vi "PDC_AVIFileSave.vi"(8 "error in (no error)":errorcluster, 9 "FrameNo":u32, 10 "ChildNo":u32, 11 "DeviceNo":u32) -> (0 "error out":errorcluster, 2 "Size":u32, 3 "ReturnValue":u32, 4 "ErrorCode":u32)   [LabVIEW 2015]
doc: "Saves AVI files for specified images which recorded by the specified child device."
uses:
  PDCLIB.dll
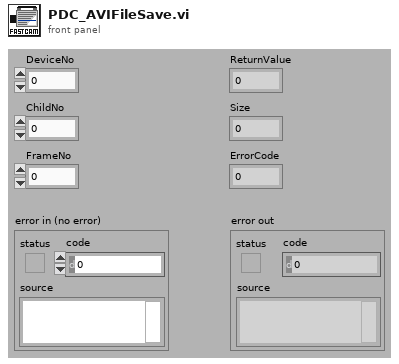
[diagram p1: front panel]
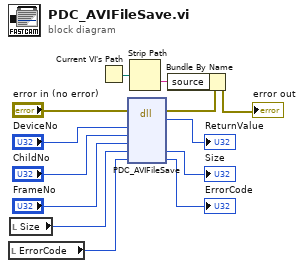
[diagram p0: block diagram]
diagram:
  n1 = local read "ErrorCode"() -> (w10:u32)
  n2 = local read "Size"() -> (w5:u32)
  n3 = Current VI's Path() -> (path=w3:path)
  n4 = dll-call lib="PDCLIB.dll" fn="PDC_AVIFileSave"(error in="error in (no error)", "nDeviceNo"="DeviceNo", "nChildNo"="ChildNo", "nFrameNo"="FrameNo", "pSize"=w5, "pErrorCode"=w10) -> (error out=w2:errorcluster, "return type"=→"ReturnValue":u32, "pSize"=→"Size":u32, "pErrorCode"=→"ErrorCode":u32)  [unwired: 5 in, 1 out]
  n5 = Strip Path(path=w3) -> (name=w4:string)  [unwired: 1 out]
  n6 = Bundle By Name(cluster=w2, "source"=w4) -> (→"error out":errorcluster)
